vi "SetChnlsOutputModuliHW.vi"(8 "error in (no error)":errorcluster, 10 "ChnlSettings":T1[](array[typedef]), 11 "BME_DG_System in":refnum<class "BME_DG_System.lvclass">) -> (0 "error out":errorcluster, 3 "BME_DG_System out":refnum<class "BME_DG_System.lvclass">)   [LabVIEW 2009, in "POLARIS BME DG.lvlib" / "BME_DG_System.lvclass"]
uses:
  BME_DG_System.lvclass
  ChnlOutputModulo.ctl
  BME_DG_Base/BME_DG_Base.lvclass
  BME_DG_Chnl/BME_DG_Chnl.lvclass
  POLARIS BME DG.lvlib
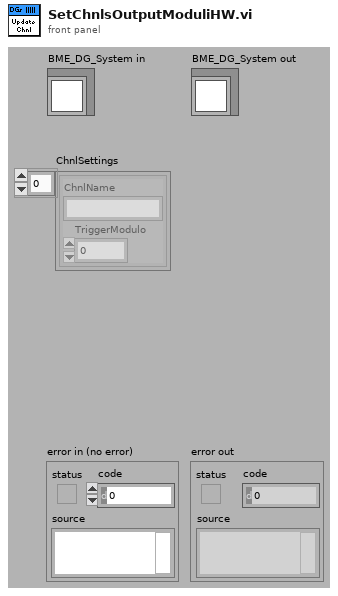
[diagram p1: front panel]
types:
  T1 = typedef "POLARIS BME DG.lvlib/ChnlOutputModulo.ctl" = cluster{"ChnlName":string, "TriggerModulo":u32}
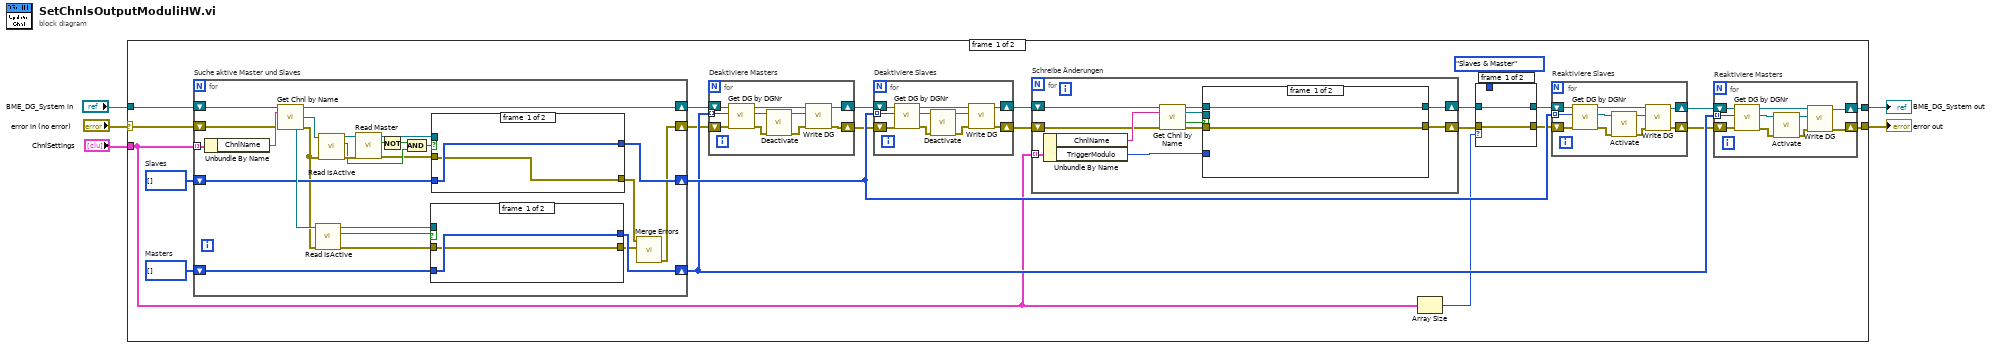
[diagram p0: block diagram]
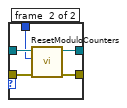
[diagram p2: hidden frame]
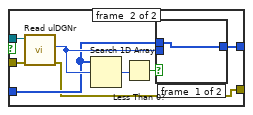
[diagram p3: hidden frame]
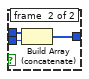
[diagram p4: hidden frame]
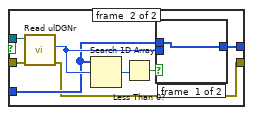
[diagram p5: hidden frame]
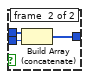
[diagram p6: hidden frame]
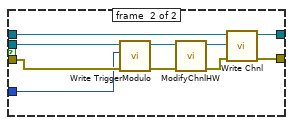
[diagram p7: hidden frame]
diagram:
  n1 = case shown="No Error" "error in (no error)" {
    selector: "error in (no error)" -> [w19 w154]
    tunnel: [w15 w154] -> w4
    tunnel: [w20 w153] -> w2
    tunnel: "BME_DG_System in" -> [w28 w153]
    tunnel: "ChnlSettings" -> [w13 _]
    frame #0 {
      w25 = u32[] []  # Slaves
      w27 = u32[] []  # Masters
      n2 = for "Suche aktive Master und Slaves" {
        tunnel: w13 -> [w99] mode=indexing
        shift-right: [w98] -> w26
        shift-left: w28 -> [w100]
        shift-right: [w96] -> w21
        shift-left: w27 -> [w97]
        shift-right: [w80] -> w23
        shift-left: w25 -> [w85]
        shift-right: [w76] -> w18
        shift-left: w19 -> [w79]
        n3 = Unbundle By Name(w99) -> ("ChnlName"=w101:string)
        n4 = call "Get Chnl by Name.vi"("BME_DG_System in"=w100, "Chnl Name"=w101, "error in (no error)"=w79) -> ("BME_DG_System out"=w98:refnum<class "BME_DG_System.lvclass">, "Owner DG"=w91:refnum<class "BME_DG_Base.lvclass">, "Master DG"=w95:refnum<class "BME_DG_Base.lvclass">, "error out"=w81:errorcluster)  [unwired: 7 in, 2 out]
        n5 = call-dynamic "Read IsActive.vi"("error in (no error)"=w81, "BME_DG_Base in"=w95) -> ("error out"=w94:errorcluster, "Active?"=w92:bool, "BME_DG_Base out"=w93:refnum<class "BME_DG_Base.lvclass">)  [unwired: 7 in]
        n6 = call-dynamic "Read IsActive.vi"("error in (no error)"=w81, "BME_DG_Base in"=w91) -> ("error out"=w89:errorcluster, "Active?"=w86:bool, "BME_DG_Base out"=w90:refnum<class "BME_DG_Base.lvclass">)  [unwired: 7 in]
        n7 = call-dynamic "Read Master.vi"("error in (no error)"=w89, "BME_DG_Base in"=w90) -> ("error out"=w82:errorcluster, "Master?"=w88:bool, "BME_DG_Base out"=w83:refnum<class "BME_DG_Base.lvclass">)  [unwired: 6 in, 1 out]
        n8 = Not(x=w88) -> (.not. x?=w87:bool)
        n9 = And(x=w87, y=w86) -> (x .and. y?=w84:bool)
        n10 = case shown="True" w92 {
          tunnel: w97 -> [w117 w122]
          tunnel: [w117 w121] -> w96
          tunnel: w94 -> [w116 w120]
          tunnel: w93 -> [_ w119]
          tunnel: [w116 w118] -> w77
          frame #0 {
          }
          frame #1 {
            n11 = call-dynamic "Read ulDGNr.vi"("error in (no error)"=w120, "BME_DG_Base in"=w119) -> ("error out"=w118:errorcluster, "ulDGNr"=w125:u32)  [unwired: 6 in, 2 out]
            n12 = Search 1D Array(1D array=w122, element=w125) -> (index of element=w124:i32)  [unwired: 1 in]
            n13 = Less Than 0?(x=w124) -> (x < 0?=w123:bool)
            n14 = case shown="True" w123 {
              tunnel: [w126 w129] -> w121
              tunnel: w125 -> [_ w128]
              tunnel: w122 -> [w126 w127]
              frame #0 {
              }
              frame #1 {
                n15 = Build Array (concatenate)(w127, w128) -> (w129:u32[])
              }
            }
          }
        }
        n16 = case shown="True" w84 {
          tunnel: w85 -> [w103 w108]
          tunnel: [w103 w107] -> w80
          tunnel: w82 -> [w102 w106]
          tunnel: w83 -> [_ w105]
          tunnel: [w102 w104] -> w78
          frame #0 {
          }
          frame #1 {
            n17 = call-dynamic "Read ulDGNr.vi"("error in (no error)"=w106, "BME_DG_Base in"=w105) -> ("error out"=w104:errorcluster, "ulDGNr"=w111:u32)  [unwired: 6 in, 2 out]
            n18 = Search 1D Array(1D array=w108, element=w111) -> (index of element=w110:i32)  [unwired: 1 in]
            n19 = Less Than 0?(x=w110) -> (x < 0?=w109:bool)
            n20 = case shown="True" w109 {
              tunnel: [w112 w115] -> w107
              tunnel: w111 -> [_ w114]
              tunnel: w108 -> [w112 w113]
              frame #0 {
              }
              frame #1 {
                n21 = Build Array (concatenate)(w113, w114) -> (w115:u32[])
              }
            }
          }
        }
        n22 = call <vilib>:"Merge Errors.vi"("error in 2 (no error)"=w77, "error in 1 (no error)"=w78) -> ("error out"=w76:errorcluster)  [unwired: 5 in]
      }
      n23 = for "Deaktiviere Masters" {
        shift-right: [w73] -> w24
        shift-left: w26 -> [w75]
        tunnel: w21 -> [w72] mode=indexing
        shift-right: [w68] -> w17
        shift-left: w18 -> [w69]
        n24 = call "Get DG by DGNr.vi"("error in (no error)"=w69, "DG Nr."=w72, "BME_DG_System in"=w75) -> ("error out"=w70:errorcluster, "BME_DG_Base.lvclass"=w71:refnum<class "BME_DG_Base.lvclass">, "BME_DG_System out"=w74:refnum<class "BME_DG_System.lvclass">)  [unwired: 5 in, 1 out]
        n25 = call-dynamic "Deactivate.vi"("error in (no error)"=w70, "BME_DG_Base in"=w71) -> ("error out"=w67:errorcluster, "BME_DG_Base out"=w66:refnum<class "BME_DG_Base.lvclass">)  [unwired: 8 in]
        n26 = call "Write DG.vi"("error in (no error)"=w67, "BME_DG_Base"=w66, "BME_DG_System in"=w74) -> ("error out"=w68:errorcluster, "BME_DG_System out"=w73:refnum<class "BME_DG_System.lvclass">)  [unwired: 7 in]
      }
      n27 = for "Deaktiviere Slaves" {
        shift-right: [w63] -> w11
        shift-left: w24 -> [w65]
        tunnel: w23 -> [w62] mode=indexing
        shift-right: [w58] -> w10
        shift-left: w17 -> [w59]
        n28 = call "Get DG by DGNr.vi"("error in (no error)"=w59, "DG Nr."=w62, "BME_DG_System in"=w65) -> ("error out"=w60:errorcluster, "BME_DG_Base.lvclass"=w61:refnum<class "BME_DG_Base.lvclass">, "BME_DG_System out"=w64:refnum<class "BME_DG_System.lvclass">)  [unwired: 5 in, 1 out]
        n29 = call-dynamic "Deactivate.vi"("error in (no error)"=w60, "BME_DG_Base in"=w61) -> ("error out"=w57:errorcluster, "BME_DG_Base out"=w56:refnum<class "BME_DG_Base.lvclass">)  [unwired: 8 in]
        n30 = call "Write DG.vi"("error in (no error)"=w57, "BME_DG_Base"=w56, "BME_DG_System in"=w64) -> ("error out"=w58:errorcluster, "BME_DG_System out"=w63:refnum<class "BME_DG_System.lvclass">)  [unwired: 7 in]
      }
      n31 = for "Schreibe Änderungen" {
        shift-right: [w135] -> w9
        shift-left: w11 -> [w136]
        tunnel: w13 -> [w134] mode=indexing
        shift-right: [w130] -> w8
        shift-left: w10 -> [w131]
        n32 = Unbundle By Name(w134) -> ("ChnlName"=w133:string, "TriggerModulo"=w132:u32)
        n33 = call "Get Chnl by Name.vi"("BME_DG_System in"=w136, "Chnl Name"=w133, "error in (no error)"=w131) -> ("BME_DG_System out"=w138:refnum<class "BME_DG_System.lvclass">, "BME_DG_Chnl"=w139:refnum<class "BME_DG_Chnl.lvclass">, "found?"=w140:bool, "error out"=w137:errorcluster)  [unwired: 7 in, 2 out]
        n34 = case shown="True" w140 {
          tunnel: w139 -> [_ w151]
          tunnel: w138 -> [w142 w145]
          tunnel: w137 -> [w141 w152]
          tunnel: [w142 w144] -> w135
          tunnel: [w141 w146] -> w130
          tunnel: w132 -> [_ w150]
          frame #0 {
          }
          frame #1 {
            n35 = call-dynamic "Write TriggerModulo.vi"("error in (no error)"=w152, "TriggerModulo"=w150, "BME_DG_G05_Chnl in"=w151) -> ("error out"=w149:errorcluster, "BME_DG_G05_Chnl out"=w148:refnum<class "BME_DG_Chnl.lvclass">)  [unwired: 7 in]
            n36 = call-dynamic "ModifyChnlHW.vi"("error in (no error)"=w149, "BME_DG_Chnl in"=w148) -> ("error out"=w147:errorcluster, "BME_DG_Chnl out"=w143:refnum<class "BME_DG_Chnl.lvclass">)  [unwired: 8 in]
            n37 = call "Write Chnl.vi"("error in (no error)"=w147, "BME_DG_Chnl.lvclass"=w143, "BME_DG_System in"=w145) -> ("error out"=w146:errorcluster, "BME_DG_System out"=w144:refnum<class "BME_DG_System.lvclass">)  [unwired: 7 in]
          }
        }
      }
      n38 = Array Size(array=w13) -> (size(s)=w14:i32)
      n39 = case shown="1, Default" w14 {
        tunnel: w9 -> [w30 w35]
        tunnel: [w30 w34] -> w7
        tunnel: w8 -> [w29 w33]
        tunnel: [w29 w32] -> w6
        tunnel: enum16{"Slaves only", "Slaves & Master"}."Slaves & Master" ("Enum") -> [_ w31]
        frame #0 {
        }
        frame #1 {
          n40 = call "ResetModuloCounters.vi"("error in (no error)"=w33, "Enum"=w31, "BME_DG_System in"=w35) -> ("error out"=w32:errorcluster, "BME_DG_System out"=w34:refnum<class "BME_DG_System.lvclass">)  [unwired: 7 in]
        }
      }
      n41 = for "Reaktiviere Slaves" {
        shift-right: [w53] -> w22
        shift-left: w7 -> [w55]
        tunnel: w23 -> [w52] mode=indexing
        shift-right: [w46] -> w16
        shift-left: w6 -> [w47]
        n42 = call "Get DG by DGNr.vi"("error in (no error)"=w47, "DG Nr."=w52, "BME_DG_System in"=w55) -> ("error out"=w48:errorcluster, "BME_DG_Base.lvclass"=w51:refnum<class "BME_DG_Base.lvclass">, "BME_DG_System out"=w54:refnum<class "BME_DG_System.lvclass">)  [unwired: 5 in, 1 out]
        n43 = call-dynamic "Activate.vi"("error in (no error)"=w48, "BME_DG_Base in"=w51) -> ("error out"=w49:errorcluster, "BME_DG_Base out"=w50:refnum<class "BME_DG_Base.lvclass">)  [unwired: 8 in]
        n44 = call "Write DG.vi"("error in (no error)"=w49, "BME_DG_Base"=w50, "BME_DG_System in"=w54) -> ("error out"=w46:errorcluster, "BME_DG_System out"=w53:refnum<class "BME_DG_System.lvclass">)  [unwired: 7 in]
      }
      n45 = for "Reaktiviere Masters" {
        shift-right: [w43] -> w20
        shift-left: w22 -> [w45]
        tunnel: w21 -> [w42] mode=indexing
        shift-right: [w36] -> w15
        shift-left: w16 -> [w37]
        n46 = call "Get DG by DGNr.vi"("error in (no error)"=w37, "DG Nr."=w42, "BME_DG_System in"=w45) -> ("error out"=w38:errorcluster, "BME_DG_Base.lvclass"=w41:refnum<class "BME_DG_Base.lvclass">, "BME_DG_System out"=w44:refnum<class "BME_DG_System.lvclass">)  [unwired: 5 in, 1 out]
        n47 = call-dynamic "Activate.vi"("error in (no error)"=w38, "BME_DG_Base in"=w41) -> ("error out"=w39:errorcluster, "BME_DG_Base out"=w40:refnum<class "BME_DG_Base.lvclass">)  [unwired: 8 in]
        n48 = call "Write DG.vi"("error in (no error)"=w39, "BME_DG_Base"=w40, "BME_DG_System in"=w44) -> ("error out"=w36:errorcluster, "BME_DG_System out"=w43:refnum<class "BME_DG_System.lvclass">)  [unwired: 7 in]
      }
    }
    frame #1 {
    }
  }
  "error out" <- w4
  "BME_DG_System out" <- w2
